vi "Cholesky Factorization Rank-1 Update_Givens Rotation (CDB).vi"(10 "b":cdb, 11 "a":cdb) -> (1 "v":cdb, 2 "s":cdb, 3 "c":dbl)   [LabVIEW 2017, in "NI_AAL_LinAlg.lvlib"]
uses:
  <vilib>/Analysis/NI_AAL_LinAlg.lvlib
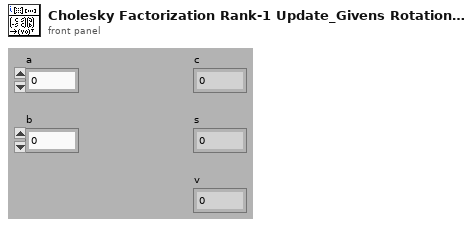
[diagram p1: front panel]
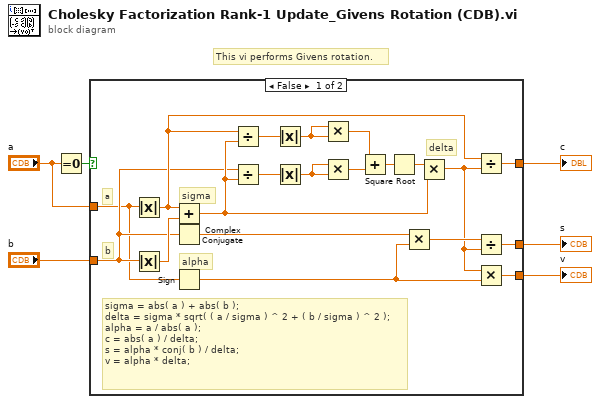
[diagram p0: block diagram]
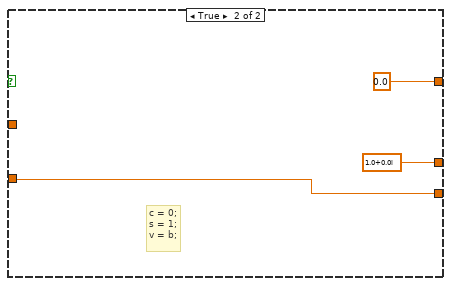
[diagram p2: hidden frame]
diagram:
  # "This vi performs Givens rotation."
  n1 = Equal To 0?(x="a") -> (x = 0?=w6:bool)
  n2 = case shown="False" w6 {
    tunnel: "b" -> [w9 w28]
    tunnel: "a" -> [w7 _]
    tunnel: [w20 0.0] -> w3
    tunnel: [w18 cdb 1.0+0.0i] -> w2
    tunnel: [w17 w28] -> w1
    frame False {
      # "alpha"
      # "b"
      # "a"
      # "delta"
      # "sigma"
      # "sigma = abs( a ) + abs( b );\ndelta = sigma * sqrt( ( a / sigma ) ^ 2 + ( b / sigma ) ^ 2 );\nalpha = a / abs( a );\nc = abs( a ) / delta;\ns = alpha * conj( b ) / delta;\nv = alpha * delta;"
      n3 = Absolute Value(x=w7) -> (abs(x)=w10:dbl)
      n4 = Absolute Value(x=w9) -> (abs(x)=w26:dbl)
      n5 = Add(x=w10, y=w26) -> (x+y=w21:dbl)
      n6 = Complex Conjugate(1:w9) -> (0:w11:cdb)
      n7 = Sign(1:w7) -> (0:w8:cdb)
      n8 = Divide(x=w10, y=w21) -> (x/y=w15:dbl)
      n9 = Divide(x=w9, y=w21) -> (x/y=w13:cdb)
      n10 = Absolute Value(x=w15) -> (abs(x)=w14:dbl)
      n11 = Absolute Value(x=w13) -> (abs(x)=w12:dbl)
      n12 = Multiply(x=w14, y=w14) -> (x*y=w24:dbl)
      n13 = Multiply(x=w12, y=w12) -> (x*y=w25:dbl)
      n14 = Add(x=w24, y=w25) -> (x+y=w23:dbl)
      n15 = Square Root(x=w23) -> (sqrt(x)=w22:dbl)
      n16 = Multiply(x=w11, y=w8) -> (x*y=w19:cdb)
      n17 = Multiply(x=w22, y=w21) -> (x*y=w16:dbl)
      n18 = Divide(x=w10, y=w16) -> (x/y=w20:dbl)
      n19 = Divide(x=w19, y=w16) -> (x/y=w18:cdb)
      n20 = Multiply(x=w16, y=w8) -> (x*y=w17:cdb)
    }
    frame True {
      # "c = 0;\ns = 1;\nv = b;"
    }
  }
  "c" <- w3
  "s" <- w2
  "v" <- w1
